vi "CRYProbe Waveform.vi"() -> ()   [LabVIEW 2013]
panel:
  out "Source Step":string caption="源步骤"
  in  "Name":string
  in  "Update?":bool
  in  "Close?":bool
  in  "Number":i32
  out "Y unit":string caption="Y轴单位"
  out "Length":string caption="时间"
  out "Fs":i32 caption="采样频率"
  out "Range":string caption="范围"
  out "WaveGraph":cluster{"xo":dbl, "dx":dbl, dbl[]}[](graph)
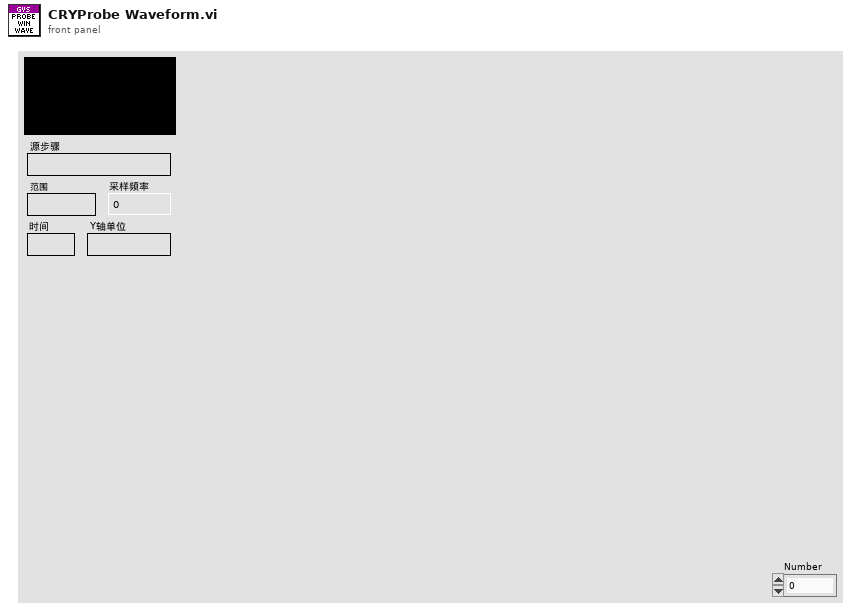
[diagram p1: front panel]
types:
  T1 = typedef "CRYWaveform Cluster.ctl" = cluster{"Waveform":cluster{"X0":dbl, "dX":dbl, "Y":sgl[]}, "X data":u16, "Y data":u16, "Y axis":u16, "X unit":string, "Y unit":string, "Y dB ref":dbl, "display Y":bool, "display X":bool, "Overload?":bool, "Test Info":string, "Step No.":i32, "Name":string, "protected":bool, "Sqc history":string[], "Signal Channel ID":i32, "Plot Settings":cluster{"Color":u32, "Interpolation":u8, "Point Style":u8, "Line Style":u8, "Point Color":u32, "Line Width":u8, "Bar Plot Style":u8, "Fill To":i16}, "AutoProtect":bool}
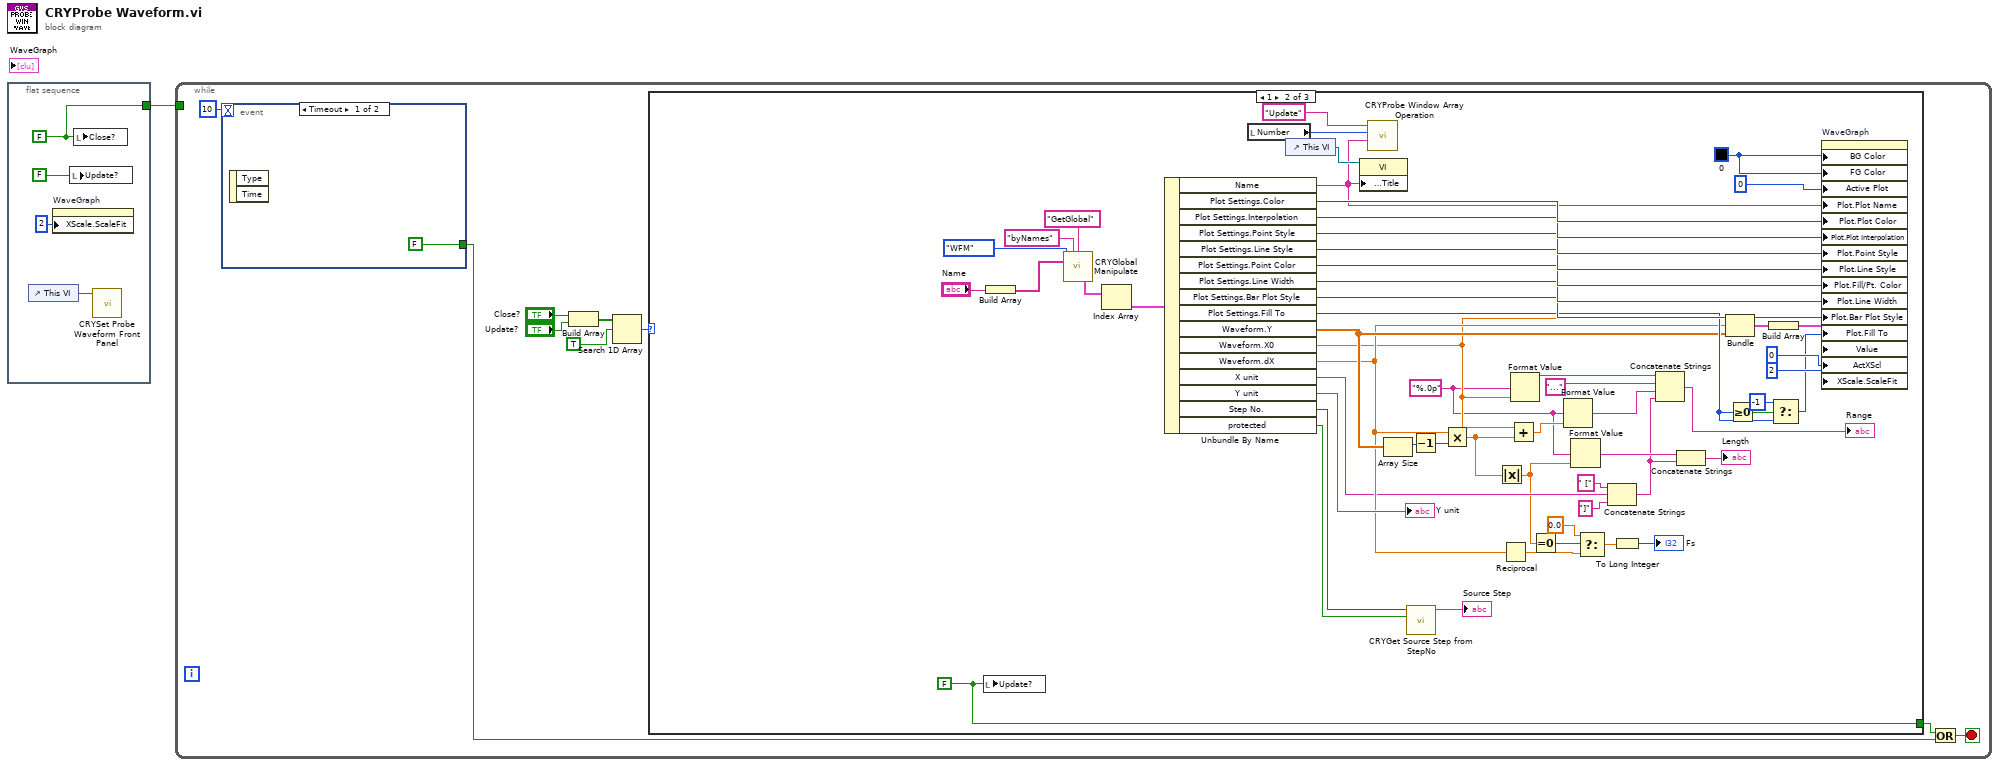
[diagram p0: block diagram]
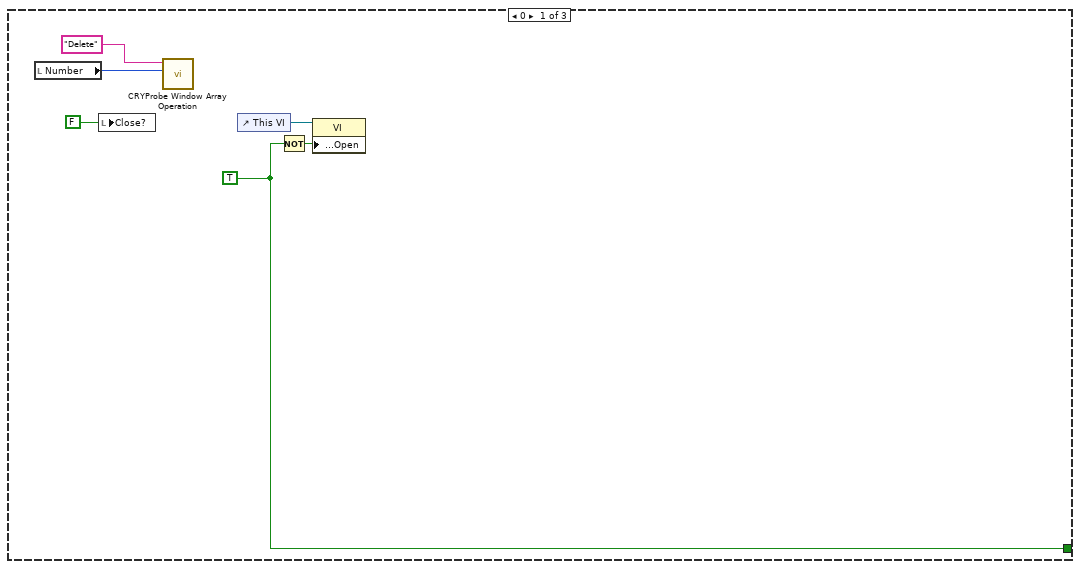
[diagram p2: hidden frame]
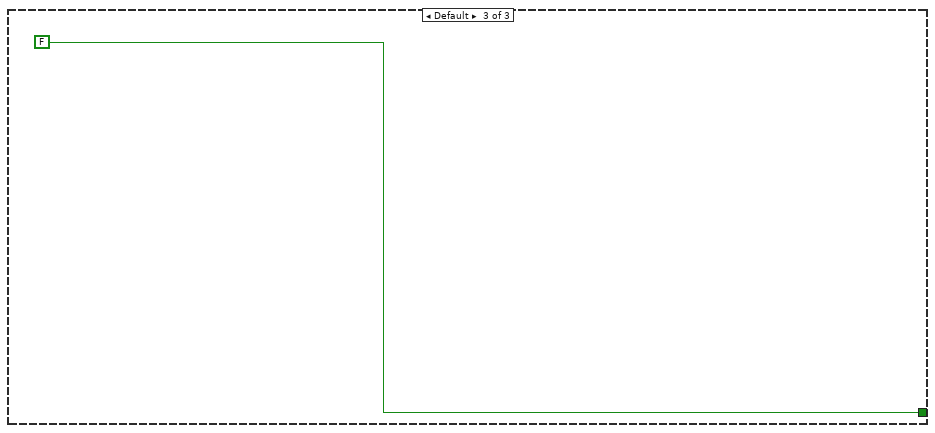
[diagram p3: hidden frame]
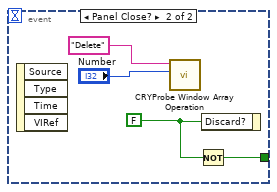
[diagram p4: hidden frame]
diagram:
  n1 = flat-sequence {
    tunnel: [w4] -> w1
    frame #0 {
      w4 = FALSE ("Close?")
      n2 = control-ref of="This VI"() -> (w2:refnum<vi>)
      n3 = property on="WaveGraph" class="WFGraph (strict)"("XScale.ScaleFit"=u8 2 ("X Scale.Scale Fit")) -> ()  [unwired: 2 in, 2 out]
      n4 = local write "Update?"(FALSE ("Close?")) -> ()
      n5 = local write "Close?"(w4) -> ()
      n6 = call "CRYSet Probe Waveform Front Panel.vi"("Vi Ref"=w2) -> ()  [unwired: 11 in]
    }
  }
  n7 = while {
    tunnel: w1 -> [_]
    stop <- w6 stop-if-true
    n8 = event shown="[0] Timeout" {
      selector: _ -> [_ _]
      dyn-events: _ -> [_ _]
      timeout: 10 -> [_ _]
      tunnel: [FALSE ("Discard?") w82] -> w7
      event Timeout {
        n9 = event-data() -> ()  [unwired: 3 out]
      }
      event Panel Close? {
        w83 = FALSE ("Discard?")
        n10 = event-data() -> ()  [unwired: 5 out]
        n11 = call "CRYProbe Window Array Operation.vi"("Number"="Number", "sAction"="Delete") -> ()  [unwired: 1 in, 9 out]
        n12 = Not(x=w83) -> (.not. x?=w82:bool)
        n13 = event-data("Discard?"=w83) -> ()  [unwired: 1 in, 1 out]
      }
    }
    n14 = Build Array("Close?", "Update?") -> (w10:bool[])
    n15 = Search 1D Array(1D array=w10, element=TRUE) -> (index of element=w11:i32)  [unwired: 1 out]
    n16 = case shown="1" w11 {
      tunnel: [w17 w72 FALSE ("Close?")] -> w8
      frame 0 {
        w17 = TRUE ("Discard?")
        n17 = local read "Number"() -> (w16:i32)
        n18 = local write "Close?"(FALSE ("Close?")) -> ()
        n19 = call "CRYProbe Window Array Operation.vi"("Number"=w16, "sAction"="Delete") -> ()  [unwired: 1 in, 9 out]
        n20 = control-ref of="This VI"() -> (w18:refnum<vi>)
        n21 = Not(x=w17) -> (.not. x?=w19:bool)
        n22 = property class="VI"(reference=w18, "Front Panel.Open"=w19) -> ()  [unwired: 1 in, 2 out]
      }
      frame 1 {
        w45 = "%.0p" ("format string")
        w72 = FALSE ("Close?")
        w73 = u32 0
        n23 = local write "Update?"(w72) -> ()
        n24 = Build Array("Name") -> (w21:string[])
        n25 = call "CRYGlobal Manipulate.vi"("Type"=enum16{"Curves", "Values", "Results", "WFM"}."WFM", "sOption"="byNames", "sAction"="GetGlobal", "sData"=w21) -> ("WFM Out"=w27:T1[])  [unwired: 5 in, 6 out]
        n26 = Index Array(array=w27) -> (element=w26:T1)  [unwired: 1 in]
        n27 = Unbundle By Name(w26) -> ("Name"=w68:string, "Plot Settings.Color"=w76:u32, "Plot Settings.Interpolation"=w74:u8, "Plot Settings.Point Style"=w65:u8, "Plot Settings.Line Style"=w64:u8, "Plot Settings.Point Color"=w63:u32, "Plot Settings.Line Width"=w62:u8, "Plot Settings.Bar Plot Style"=w61:u8, "Plot Settings.Fill To"=w56:i16, "Waveform.Y"=w48:sgl[], "Waveform.X0"=w46:dbl, "Waveform.dX"=w47:dbl, "X unit"=w42:string, "Y unit"=→"Y unit":string, "Step No."=w30:i32, "protected"=w29:bool)
        n28 = local read "Number"() -> (w67:i32)
        n29 = control-ref of="This VI"() -> (w77:refnum<vi>)
        n30 = property class="VI"(reference=w77, "Front Panel.Title"=w68) -> ()  [unwired: 1 in, 2 out]
        n31 = call "CRYProbe Window Array Operation.vi"("Name"=w68, "Number"=w67, "sAction"="Update") -> ()  [unwired: 9 out]
        n32 = Array Size(array=w48) -> (size(s)=w50:i32)
        n33 = call "CRYGet Source Step from StepNo.vi"("Protect?"=w29, "Step No."=w30) -> ("StepName"=→"Source Step":string)  [unwired: 9 in]
        n34 = Decrement(x=w50) -> (x-1=w31:i32)
        n35 = Multiply(x=w47, y=w31) -> (x*y=w32:dbl)
        n36 = Absolute Value(x=w32) -> (abs(x)=w37:dbl)
        n37 = Reciprocal(x=w47) -> (1/x=w35:dbl)
        n38 = Add(x=w46, y=w32) -> (x+y=w54:dbl)
        n39 = Format Value(format string=w45, value (0)=w46) -> (output string=w53:string)  [unwired: 1 in]
        n40 = Equal To 0?(x=w37) -> (x = 0?=w36:bool)
        n41 = Format Value(format string=w45, value (0)=w54) -> (output string=w51:string)  [unwired: 1 in]
        n42 = Format Value(format string=w45, value (0)=w37) -> (output string=w41:string)  [unwired: 1 in]
        n43 = Select(t=0.0, s=w36, f=w35) -> (s? t:f=w33:dbl)
        n44 = Concatenate Strings(" [", w42, "]") -> (w40:string)
        n45 = To Long Integer(number=w33) -> (32bit integer=→"Fs":i32)
        n46 = Concatenate Strings(w53, "...", w51, w40) -> (→"Range":string)
        n47 = Concatenate Strings(w41, w40) -> (→"Length":string)
        n48 = Bundle("X0"=w46, "dX"=w47, "Y"=w48) -> (w60:cluster{"X0":dbl, "dX":dbl, "Y":sgl[]})  [unwired: 1 in]
        n49 = Greater Or Equal To 0?(x=w56) -> (x >= 0?=w57:bool)
        n50 = Build Array(w60) -> (w59:cluster{"X0":dbl, "dX":dbl, "Y":sgl[]}[])
        n51 = Select(t=i16 -1 ("Fill To"), s=w57, f=w56) -> (s? t:f=w55:i16)
        n52 = property on="WaveGraph" class="WFGraph (strict)"("BG Color"=w73, "FG Color"=w73, "Active Plot"=u32 0, "Plot.Plot Name"=w68, "Plot.Plot Color"=w76, "Plot.Plot Interpolation"=w74, "Plot.Point Style"=w65, "Plot.Line Style"=w64, "Plot.Fill/Pt. Color"=w63, "Plot.Line Width"=w62, "Plot.Bar Plot Style"=w61, "Plot.Fill To"=w55, "Value"=w59, "ActXScl"=0 ("Active X Scale"), "XScale.ScaleFit"=u8 2 ("X Scale.Scale Fit")) -> ()  [unwired: 2 in, 2 out]
      }
      frame Default {
      }
    }
    n53 = Or(x=w8, y=w7) -> (x .or. y?=w6:bool)
  }
